vi "GetParam.vi"(8 "error in (no error)":errorcluster caption="entrée d'erreur (pas d'erreur)", 11 "normalize.lvclass":refnum<class "normalize.lvclass">) -> (0 "error out":errorcluster caption="sortie d'erreur", 2 "normalize":T1={"norm"="l2", "axis"=1, "copy"=TRUE, "Returns"="X"}, 3 "normalize.lvclass":refnum<class "normalize.lvclass">)   [LabVIEW 2020, in "normalize.lvclass"]
doc: "Get Parameters"
uses:
  normalize.lvclass
  normalize.lvclass/normalize.ctl
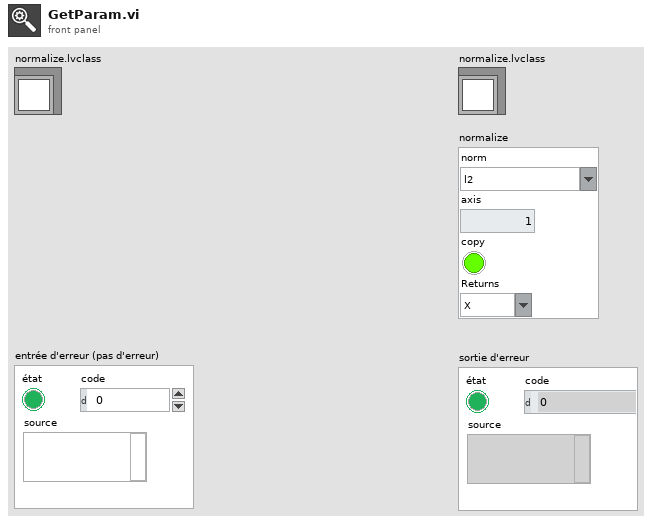
[diagram p1: front panel]
types:
  T1 = cluster{"norm":string, "axis":i32, "copy":bool, "Returns":string}
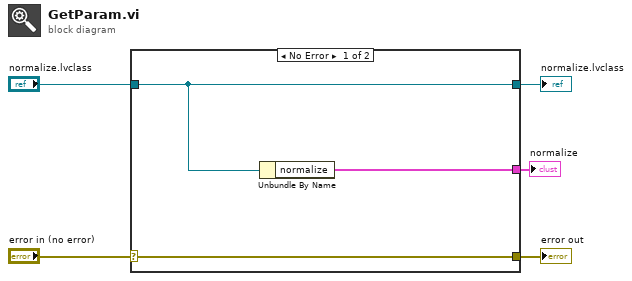
[diagram p0: block diagram]
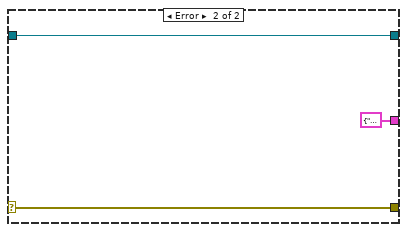
[diagram p2: hidden frame]
diagram:
  n1 = case shown="No Error" "error in (no error)" {
    selector: "error in (no error)" -> [w8 w10]
    tunnel: [w8 w10] -> w4
    tunnel: [w7 w11] -> w2
    tunnel: "normalize.lvclass" -> [w7 w11]
    tunnel: [w6 T1 {"norm"="", "axis"=0, "copy"=FALSE, "Returns"=""} ("normalize")] -> w1
    frame No Error {
      n2 = Unbundle By Name(w7) -> ("normalize"=w6:T1)
    }
    frame Error {
    }
  }
  "error out" <- w4
  "normalize.lvclass" <- w2
  "normalize" <- w1
